vi "image properties.vi"(0 "Image in":T1, 5 "error in (no error)":errorcluster) -> (13 "Image Name":string, 14 "Image out":T1, 15 "Pixel Pointer out":u64, 16 "Line Width":i32, 17 "X Resolution":i32, 18 "Y Resolution":i32, 19 "error out":errorcluster)   [LabVIEW 2017, in "Vision.lvlib"]
uses:
  Vision.lvlib
  <vilib>/vision/Image Controls.llb/IMAQ Image.ctl
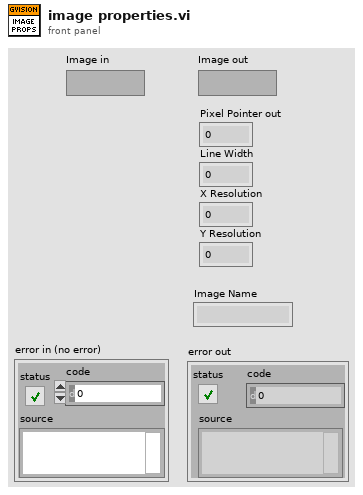
[diagram p1: front panel]
types:
  T1 = typedef "IMAQ Image.ctl" = refnum<image>
  T2 = enum32{"Map Pixel Pointer", "Unmap Pixel Pointer", "Get Pixels Infos"}
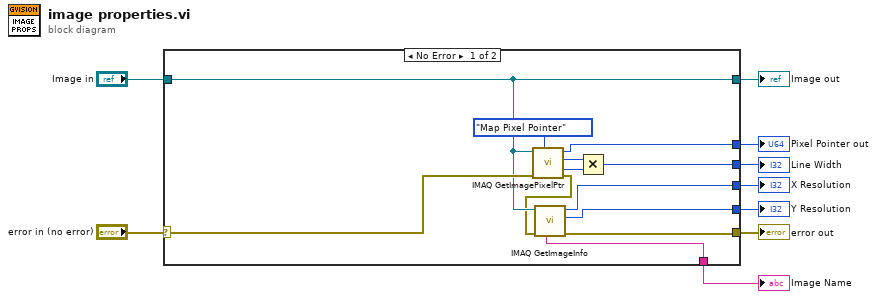
[diagram p0: block diagram]
diagram:
  n1 = case shown="No Error" "error in (no error)" {
    selector: "error in (no error)" -> [w18 w23]
    tunnel: "Image in" -> [w15 w22]
    tunnel: [w11 w23] -> w7
    tunnel: [w15 w22] -> w6
    tunnel: [w17 _] -> w5
    tunnel: [w16 _] -> w4
    tunnel: [w13 _] -> w3
    tunnel: [w12 _] -> w2
    tunnel: [w10 _] -> w1
    frame No Error {
      n2 = call "IMAQ GetImagePixelPtr"("Function"=T2."Map Pixel Pointer", "error in (no error)"=w18, "Image"=w15) -> ("error out"=w14:errorcluster, "Pixel Size (Bytes)"=w19:i32, "LineWidth(Pixels)"=w20:i32, "Pixel Pointer out"=w17:u64)  [unwired: 3 in, 2 out]
      n3 = call "IMAQ GetImageInfo"("error in (no error)"=w14, "Image"=w15) -> ("error out"=w11:errorcluster, "Y Resolution"=w12:i32, "X Resolution"=w13:i32, "Image Name"=w10:string)  [unwired: 2 in, 4 out]
      n4 = Multiply(x=w20, y=w19) -> (x*y=w16:i32)
    }
    frame Error {
    }
  }
  "Image out" <- w6
  "error out" <- w7
  "Pixel Pointer out" <- w5
  "Line Width" <- w4
  "X Resolution" <- w3
  "Y Resolution" <- w2
  "Image Name" <- w1
